vi "Read Path.vi"() -> (3 "all rows":dbl[][](array[numeric]))   [LabVIEW 2020]
uses:
  Framework/Robot Global Data.vi
  <vilib>/Utility/file.llb/Read Delimited Spreadsheet (DBL).vi
panel:
  out "path":path
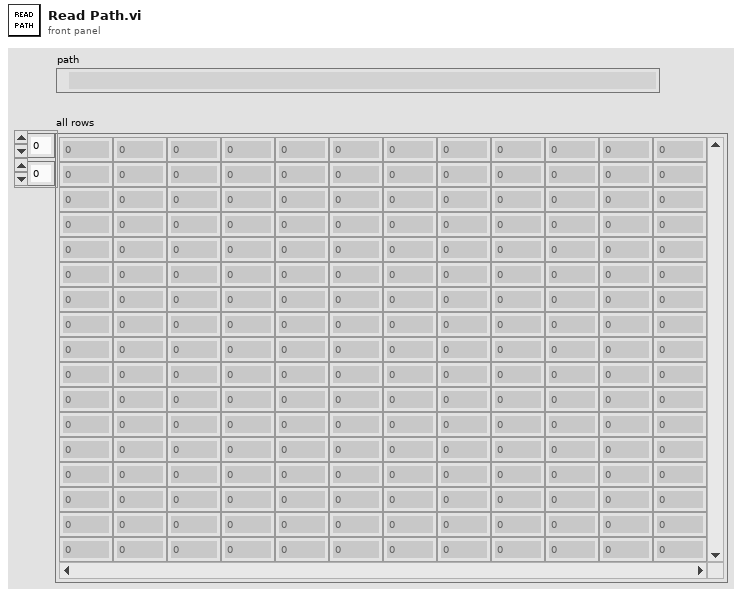
[diagram p1: front panel]
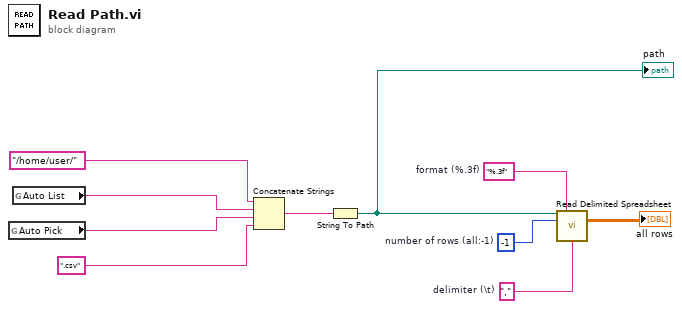
[diagram p0: block diagram]
diagram:
  w7 = -1  # number of rows (all:-1)
  w10 = "%.3f"  # format (%.3f)
  w9 = ","  # delimiter (\t)
  n1 = global read "Robot Global Data.vi" "Auto Pick"() -> (w6:string)
  n2 = global read "Robot Global Data.vi" "Auto List"() -> (w5:string)
  n3 = Concatenate Strings("/home/user/", w5, w6, ".csv") -> (w4:string)
  n4 = String To Path(string=w4) -> (path=w1:path)
  "path" <- w1
  n5 = call-poly <vilib>:"Read Delimited Spreadsheet.vi"("file path (dialog if empty)"=w1, "format (%.3f)"=w10, "number of rows (all:-1)"=w7, "delimiter (\\t)"=w9) -> ("all rows"=→"all rows":dbl[][])  [unwired: 6 in, 5 out]
